vi "Check&RPN.vi"(8 "error in (no error)":errorcluster, 11 "Array Parsed Expression":T1[](array[typedef])) -> (0 "error out":errorcluster, 3 "Array Parsed Expression":T1[](array[typedef]))   [LabVIEW 2014, in "MathProg.lvlib"]
doc: "Chequea Sintaxis y convierte a RPN."
uses:
  MathProg.lvlib
  TypeDefs/ParsedExpression.ctl
  TypeDefs/typeMed.ctl
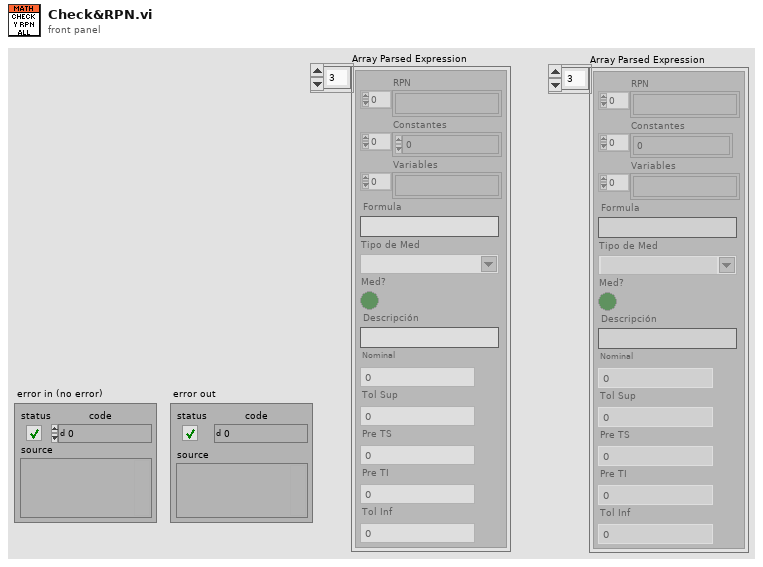
[diagram p1: front panel]
types:
  T1 = typedef "MathProg.lvlib/ParsedExpression.ctl" = cluster{"RPN ":string[], "Constantes":sgl[], "Variables":string[], "Formula":string, "Tipo de Med":T2, "Med?":bool, "Descripción":string, "Nominal":sgl, "Tol Sup":sgl, "Pre TS":sgl, "Pre TI":sgl, "Tol Inf":sgl}
  T2 = typedef "MathProg.lvlib/typeMed.ctl" = string
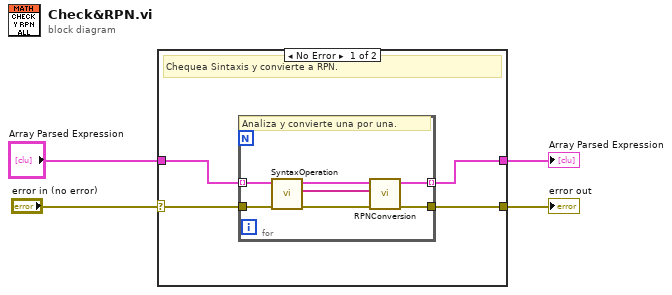
[diagram p0: block diagram]
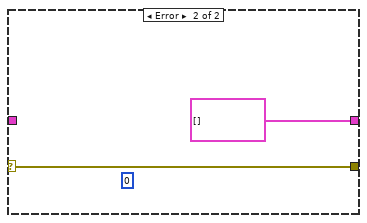
[diagram p2: hidden frame]
diagram:
  n1 = case shown="No Error" "error in (no error)" {
    selector: "error in (no error)" -> [w6 w17]
    tunnel: [w5 T1[] []] -> w4
    tunnel: [w7 w17] -> w3
    tunnel: "Array Parsed Expression" -> [w8 _]
    frame No Error {
      # "Chequea Sintaxis y convierte a RPN."
      n2 = for {
        tunnel: w8 -> [w15] mode=indexing
        tunnel: [w14] -> w5 mode=indexing
        tunnel: [w13] -> w7
        tunnel: w6 -> [w12]
        # "Analiza y convierte una por una."
        n3 = call "SyntaxOperation.vi"("error in (no error)"=w12, "Parsed Expression In"=w15) -> ("error out"=w9:errorcluster, "Token"=w10:string[], "Parsed Expression Out"=w11:T1)  [unwired: 6 in, 1 out]
        n4 = call "RPNConversion.vi"("error in"=w9, "Token"=w10, "Parsed Expression In"=w11) -> ("error out"=w13:errorcluster, "Parsed Expression Out"=w14:T1)  [unwired: 7 in]
      }
    }
    frame Error {
      (unwired) 0 ("Error Index Out")
    }
  }
  "error out" <- w3
  "Array Parsed Expression" <- w4
